vi "tqxcxtformation.vi"(0 "object in":refnum<class "212format_work.lvclass">, 1 "in":T1, 5 "error in (no error)":errorcluster) -> (14 "object out":refnum<class "212format_work.lvclass">, 15 "out":T2, 19 "error out":errorcluster)   [LabVIEW 2016, in "212format_work.lvclass"]
uses:
  212format_work.lvclass
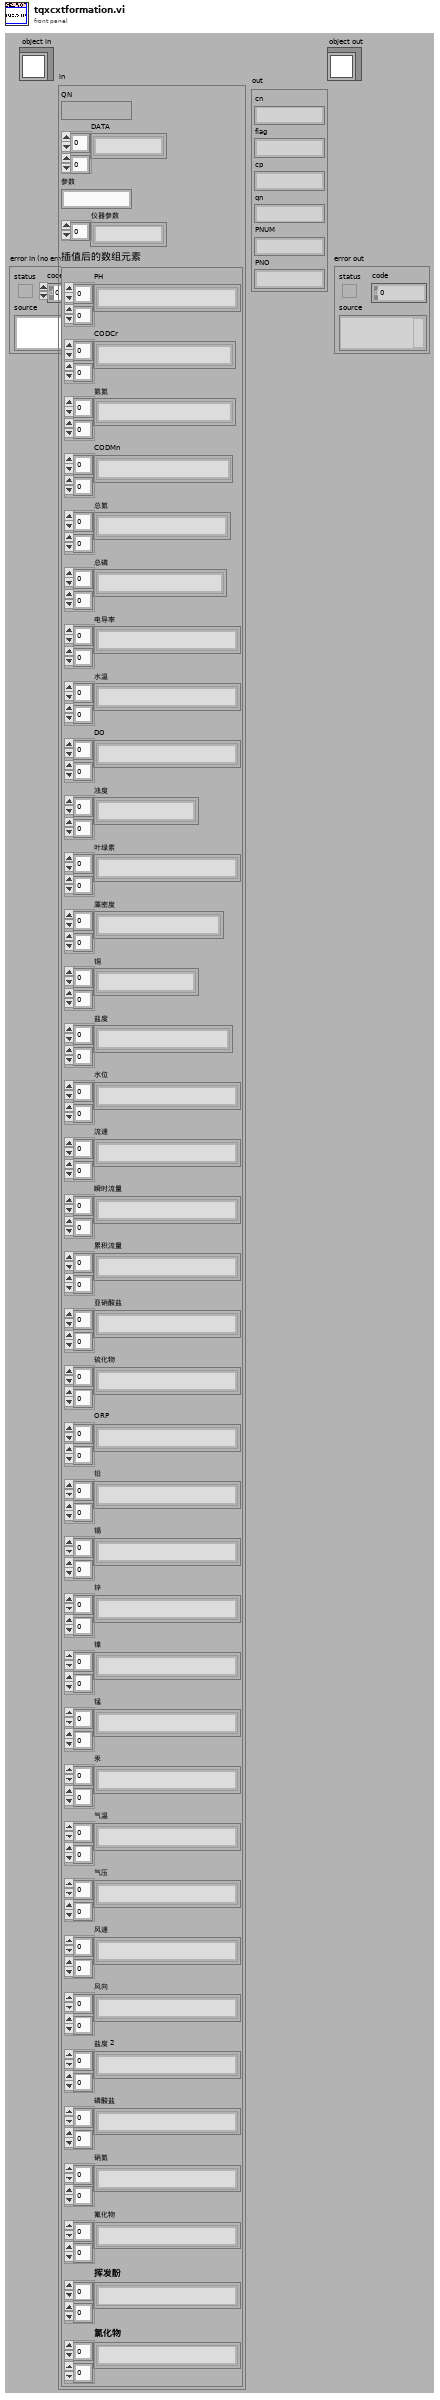
[diagram p1: front panel]
types:
  T1 = cluster{"QN":string, "DATA":string[][], "参数":string, "仪器参数":string[], "插值后的数组元素":cluster{"PH":string[][], "CODCr":string[][], "氨氮":string[][], "CODMn":string[][], "总氮":string[][], "总磷":string[][], "电导率":string[][], "水温":string[][], "DO":string[][], "浊度":string[][], "叶绿素":string[][], "藻密度":string[][], "铜":string[][], "盐度":string[][], "水位":string[][], "流速":string[][], "瞬时流量":string[][], "累积流量":string[][], "亚硝酸盐":string[][], "硫化物":string[][], "ORP":string[][], "铅":string[][], "镉":string[][], "锌":string[][], "镍":string[][], "锰":string[][], "汞":string[][], "气温":string[][], "气压":string[][], "风速":string[][], "风向":string[][], "盐度 2":string[][], "磷酸盐":string[][], "硝氮":string[][], "氟化物":string[][], "挥发酚":string[][], "氯化物":string[][]}}
  T2 = cluster{"cn":string, "flag":string, "cp":string, "qn":string, "PNUM":string, "PNO":string}
  T3 = typedef "212format_work.lvclass/interdata控件.ctl" = cluster{"数据发送协议":enum16{"2005-212协议", "2017-212协议"}, "枚举":enum16{"返回请求应答", "上传数据", "返回执行结果"}, "系统编码ST":string, "主动上报数据中":bool, "数据组合发送":bool, "地表水/污染源":bool, "应用环境":enum16{"STD", "GB212"}}
  T4 = typedef "212format_work.lvclass/data控件.ctl" = cluster{"选择发送的参数":string, "插值后的数组元素":cluster{"PH":string[][], "CODCr":string[][], "氨氮":string[][], "CODMn":string[][], "总氮":string[][], "总磷":string[][], "电导率":string[][], "水温":string[][], "DO":string[][], "浊度":string[][], "叶绿素":string[][], "藻密度":string[][], "铜":string[][], "盐度":string[][], "水位":string[][], "流速":string[][], "瞬时流量":string[][], "累积流量":string[][], "亚硝酸盐":string[][], "硫化物":string[][], "ORP":string[][], "铅":string[][], "镉":string[][], "锌":string[][], "镍":string[][], "锰":string[][], "汞":string[][], "气温":string[][], "气压":string[][], "风速":string[][], "风向":string[][], "盐度 2":string[][], "磷酸盐":string[][], "硝氮":string[][], "氟化物":string[][], "挥发酚":string[][], "氯化物":string[][]}, "register values":u16[], "columns输出":string[], "环境参数":string[][], "仪器编码":string, "实时数据发送间隔":u32, "实时数据参数":string, "参数系数簇":cluster{"CODMn":dbl, "CODCr":dbl, "DO":dbl, "铜":dbl, "PH":dbl, "氨氮":dbl, "比电导率":dbl, "水温":dbl, "COD":dbl, "浊度":dbl, "总氮":dbl, "总磷":dbl, "叶绿素a":dbl, "藻密度":dbl, "水位":dbl, "流速":dbl, "瞬时流量":dbl, "累积流量":dbl, "亚硝酸盐":dbl, "硫化物":dbl, "ORP":dbl, "铅":dbl, "镉":dbl, "锌":dbl, "镍":dbl, "锰":dbl, "汞":dbl, "气温":dbl, "气压":dbl, "风速":dbl, "风向":dbl, "盐度":dbl, "磷酸盐":dbl, "硝氮":dbl, "氟化物":dbl, "挥发酚":dbl, "氯化物":dbl}, "因子编码簇":cluster{"CODMn":string, "CODCr":string, "DO":string, "铜":string, "PH":string, "氨氮":string, "比电导率":string, "水温":string, "COD":string, "浊度":string, "总氮":string, "总磷":string, "叶绿素a":string, "藻密度":string, "水位":string, "流速":string, "瞬时流量":string, "累积流量":string, "亚硝酸盐":string, "硫化物":string, "ORP":string, "铅":string, "镉":string, "锌":string, "镍":string, "锰":string, "汞":string, "气温":string, "气压":string, "风速":string, "风向":string, "盐度":string, "磷酸盐":string, "硝氮":string, "氟化物":string, "挥发酚":string, "氯化物":string}, "小时数据发送次数":i32, "读取试剂余量的值":u16[], "参数编码":string, "数据数组大小":i32, "总包数":i32, "当前包号":i32, "columns":string[], "剖面多参数":string[][], "分包标准":i32}
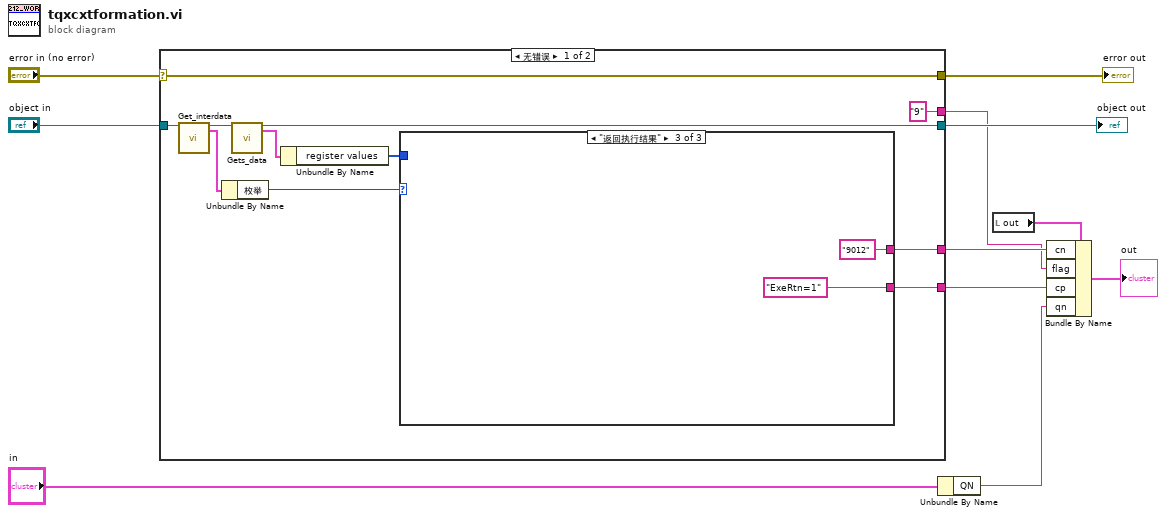
[diagram p0: block diagram]
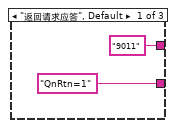
[diagram p2: hidden frame]
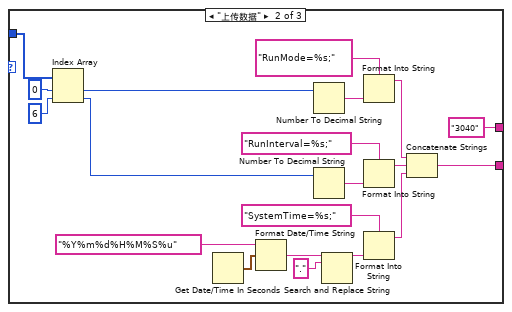
[diagram p3: hidden frame]
diagram:
  n1 = case shown="无错误" "error in (no error)" {
    selector: "error in (no error)" -> [w22 w48]
    tunnel: [w22 w48] -> w10
    tunnel: [w15 w47] -> w8
    tunnel: "object in" -> [w20 w47]
    tunnel: [w13 _] -> w3
    tunnel: [w17 _] -> w5
    tunnel: ["9" ("ST") _] -> w4
    frame No Error {
      n2 = call-dynamic "Get_interdata.vi"("object in"=w20) -> ("object out"=w16:refnum<class "212format_work.lvclass">, "interdata"=w19:T3)  [unwired: 16 in, 1 out]
      n3 = Unbundle By Name(w19) -> ("枚举"=w18:enum16{"返回请求应答", "上传数据", "返回执行结果"})
      n4 = call-dynamic "Gets_data.vi"("object in"=w16) -> ("object out"=w15:refnum<class "212format_work.lvclass">, "data"=w14:T4)  [unwired: 16 in, 1 out]
      n5 = Unbundle By Name(w14) -> ("register values"=w12:u16[])
      n6 = case shown="\"返回执行结果\"" w18 {
        tunnel: ["9011" ("CN") "3040" ("CN") "9012" ("CN")] -> w17
        tunnel: ["QnRtn=1" w26 "ExeRtn=1"] -> w13
        tunnel: w12 -> [_ w25 _]
        frame "返回请求应答", Default {
        }
        frame "上传数据" {
          n7 = Index Array(array=w25, index #1=0 ("索引"), index #2=6 ("索引")) -> (element #1=w40:u16, element #2=w27:u16)
          n8 = Get Date/Time In Seconds() -> (seconds since 1Jan1904=w30:timestamp)
          n9 = Format Date/Time String(time format string (%c)="%Y%m%d%H%M%S%u" ("时间格式字符串(%c)"), seconds (now)=w30) -> (date/time string=w33:string)  [unwired: 1 in]
          n10 = Number To Decimal String(number=w40) -> (decimal integer string=w42:string)  [unwired: 1 in]
          n11 = Number To Decimal String(number=w27) -> (decimal integer string=w36:string)  [unwired: 1 in]
          n12 = Search and Replace String(input string=w33, search string="." ("搜索字符串")) -> (result string=w29:string)  [unwired: 6 in, 3 out]
          n13 = Format Into String(format string="RunMode=%s;" ("格式字符串"), w42) -> (resulting string=w39:string)  [unwired: 2 in, 1 out]
          n14 = Format Into String(format string="RunInterval=%s;" ("格式字符串"), w36) -> (resulting string=w37:string)  [unwired: 2 in, 1 out]
          n15 = Format Into String(format string="SystemTime=%s;" ("格式字符串"), w29) -> (resulting string=w34:string)  [unwired: 2 in, 1 out]
          n16 = Concatenate Strings(w39, w37, w34) -> (w26:string)
        }
        frame "返回执行结果" {
        }
      }
    }
    frame Error {
    }
  }
  "error out" <- w10
  "object out" <- w8
  n17 = Unbundle By Name("in") -> ("QN"=w1:string)
  n18 = local read "out"() -> (w7:T2)
  n19 = Bundle By Name(cluster=w7, "cn"=w5, "flag"=w4, "cp"=w3, "qn"=w1) -> (→"out":T2)
